vi "Close.vi"(8 "error in (no error)":errorcluster, 11 "Driver in":refnum<class "Driver.lvclass">) -> (0 "error out":errorcluster, 3 "Driver out":refnum<class "Driver.lvclass">)   [LabVIEW 2023, in "HAF.lvlib" / "Driver.lvclass"]
doc: "Close the Driver ensuring a clean disconnect/tidyup of Resource connections."
uses:
  Driver.lvclass
  Driver.lvclass/Driver.ctl
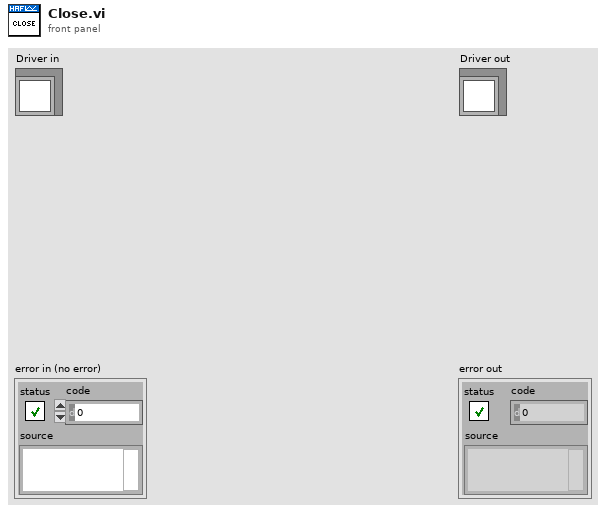
[diagram p1: front panel]
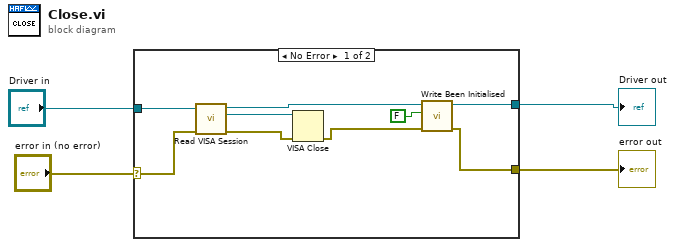
[diagram p0: block diagram]
diagram:
  n1 = case shown="No Error" "error in (no error)" {
    selector: "error in (no error)" -> [w12 w15]
    tunnel: [w6 w15] -> w3
    tunnel: [w5 w14] -> w1
    tunnel: "Driver in" -> [w13 w14]
    frame No Error {
      n2 = call-dynamic "Read VISA Session.vi"("error in (no error)"=w12, "Driver in"=w13) -> ("error out"=w10:errorcluster, "VISA Session"=w11:refnum<visa-resource-name>, "Driver out"=w9:refnum<class "Driver.lvclass">)  [unwired: 7 in]
      n3 = VISA Close(VISA resource name=w11, error in (no error)=w10) -> (error out=w8:errorcluster)
      n4 = call-dynamic "Write Been Initialised.vi"("error in (no error)"=w8, "Been Initialised"=FALSE, "Driver in"=w9) -> ("error out"=w6:errorcluster, "Driver out"=w5:refnum<class "Driver.lvclass">)  [unwired: 7 in]
    }
    frame Error {
    }
  }
  "error out" <- w3
  "Driver out" <- w1
